vi "Initialize EtherCAT youBot Gripper.vi"(8 "error in (no error)":errorcluster, 11 "gripper slave info in":T1 {"nodeAddr" format="%.0x"}) -> (0 "error out":errorcluster, 3 "KUKA youBot gripper_EtherCAT out":refnum<class "NI_Robotics_KUKA youBot Gripper_EtherCAT.lvclass">)   [LabVIEW 2017, in "NI_Robotics_KUKA youBot Host.lvlib" / "NI_Robotics_KUKA youBot Gripper_EtherCAT.lvclass"]
uses:
  <vilib>/robotics/KUKA youBot/Basic Device/Gripper EtherCAT/NI_Robotics_KUKA youBot Gripper_EtherCAT.lvclass
  c:/Program Files (x86)/National Instruments/LabVIEW 2017/vi.lib/robotics/KUKA youBot/Basic Device/Gripper/NI_Robotics_KUKA youBot Gripper.lvclass
  <vilib>/robotics/KUKA youBot/EtherCAT/Motor Slave Info.ctl
  <vilib>/robotics/KUKA youBot/EtherCAT/LowLevel/Mater Handler.ctl
  <vilib>/robotics/KUKA youBot/Motor/Gripper Motor EtherCAT/Gripper Motor Param.ctl
  <vilib>/robotics/KUKA youBot/Motor/Gripper Motor EtherCAT/NI_Robotics_KUKA youBot Gripper Motor_EtherCAT.lvclass
  c:/Program Files (x86)/National Instruments/LabVIEW 2017/vi.lib/robotics/KUKA youBot/Motor/Gripper Motor/NI_Robotics_KUKA youBot Gripper Motor.lvclass
  <vilib>/robotics/KUKA youBot/Basic Device/Gripper/NI_Robotics_KUKA youBot Gripper.lvclass
  <vilib>/robotics/KUKA youBot/NI_Robotics_KUKA youBot Host.lvlib
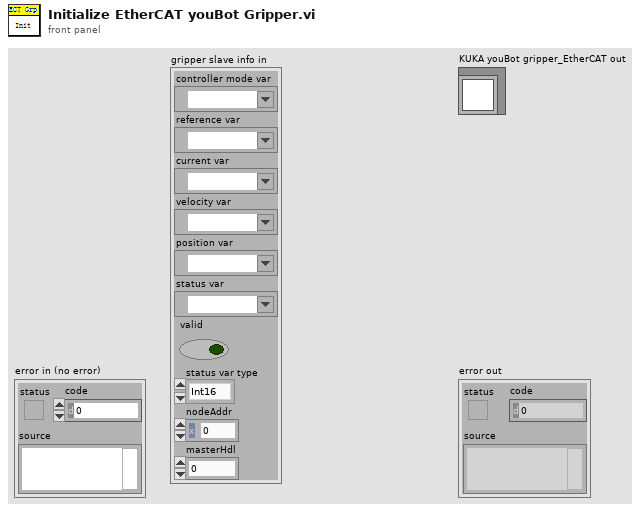
[diagram p1: front panel]
types:
  T1 = typedef "NI_Robotics_KUKA youBot Host.lvlib/Motor Slave Info.ctl" = cluster{"controller mode var":refnum<k21>, "reference var":refnum<k21>, "current var":refnum<k21>, "velocity var":refnum<k21>, "position var":refnum<k21>, "status var":refnum<k21>, "valid":bool, "status var type":enum16{"Int16", "Int32"}, "nodeAddr":u16, "masterHdl":T2}
  T2 = typedef "NI_Robotics_KUKA youBot Host.lvlib/Mater Handler.ctl" = i32
  T3 = typedef "NI_Robotics_KUKA youBot Host.lvlib/NI_Robotics_KUKA youBot Gripper Motor_EtherCAT.lvclass/Gripper Motor Param.ctl" = cluster{"ticks per meter":dbl, "ticks offset":i32, "StallGuard2Threshold":dbl, "StallGuard2FilterEnable":bool, "do calibration?":bool, "positive calibtration direction?":bool, "calibration max current (A)":dbl}
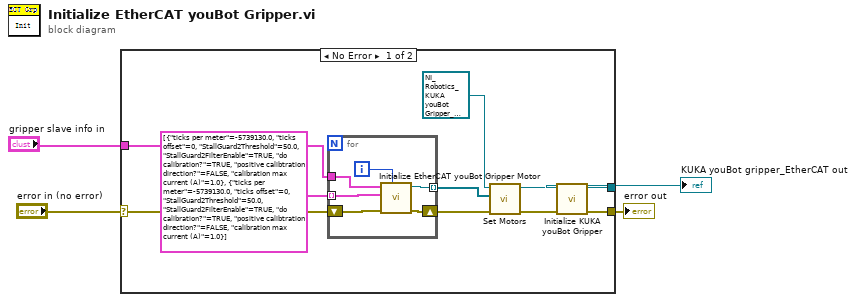
[diagram p0: block diagram]
diagram:
  n1 = case shown="No Error" "error in (no error)" {
    selector: "error in (no error)" -> [w12 w21]
    tunnel: [w7 w21] -> w3
    tunnel: "gripper slave info in" -> [w14 _]
    tunnel: [w5 _] -> w2
    frame No Error {
      n2 = for {
        tunnel: w14 -> [w20]
        tunnel: T3[] [{"ticks per meter"=-5739130.0, "ticks offset"=0, "StallGuard2Threshold"=50.0, "StallGuard2FilterEnable"=TRUE, "do calibration?"=TRUE, "positive calibtration direction?"=FALSE, "calibration max current (A)"=1.0}, {"ticks per meter"=-5739130.0, "ticks offset"=0, "StallGuard2Threshold"=50.0, "StallGuard2FilterEnable"=TRUE, "do calibration?"=TRUE, "positive calibtration direction?"=FALSE, "calibration max current (A)"=1.0}] -> [w19] mode=indexing
        shift-right: [w17] -> w11
        shift-left: w12 -> [w18]
        tunnel: [w15] -> w10 mode=indexing
        i -> [w16]
        n3 = call <vilib>:"Initialize EtherCAT youBot Gripper Motor.vi"("index"=w16, "error in (no error)"=w18, "gripper motor param"=w19, "motor slave info in"=w20) -> ("error out"=w17:errorcluster, "KUKA youBot gripper motor_EtherCAT out"=w15:refnum<class "NI_Robotics_KUKA youBot Gripper Motor_EtherCAT.lvclass">)  [unwired: 6 in]
      }
      n4 = call-dynamic "Set Motors.vi"("error in (no error)"=w11, "motors"=w10, "KUKA youBot gripper in"=refnum<class "NI_Robotics_KUKA youBot Gripper_EtherCAT.lvclass"> refnum ("NI_Robotics_KUKA youBot Host.lvlib:NI_Robotics_KUKA youBot Gripper_EtherCAT.lvclass")) -> ("error out"=w8:errorcluster, "KUKA youBot gripper out"=w6:refnum<class "NI_Robotics_KUKA youBot Gripper_EtherCAT.lvclass">)  [unwired: 7 in]
      n5 = call <vilib>:"Initialize KUKA youBot Gripper.vi"("error in (no error)"=w8, "KUKA youBot gripper in"=w6) -> ("error out"=w7:errorcluster, "KUKA youBot gripper out"=w5:refnum<class "NI_Robotics_KUKA youBot Gripper_EtherCAT.lvclass">)  [unwired: 8 in]
    }
    frame Error {
    }
  }
  "error out" <- w3
  "KUKA youBot gripper_EtherCAT out" <- w2
